vi "InitCell.vi"(6 "Color":u32, 7 "HeadPos":T1, 8 "error in (no error)":errorcluster, 9 "Direction":T2, 10 "CellPosInBody":u16, 11 "Cell":enum16{"Head", "Tail", "Body"}(ring)) -> (0 "error out":errorcluster, 3 "SnakeBodyCell out":refnum<class "SnakeBodyCell.lvclass">)   [LabVIEW 2018, in "SnakeBodyCell.lvclass"]
uses:
  SnakeBodyCell.lvclass
  Typedefs/UnitDirection.ctl
  Typedefs/XYposition.ctl
  SnakeBodyCell.lvclass/SnakeBodyCell.ctl
panel:
  # "Connector Pane"
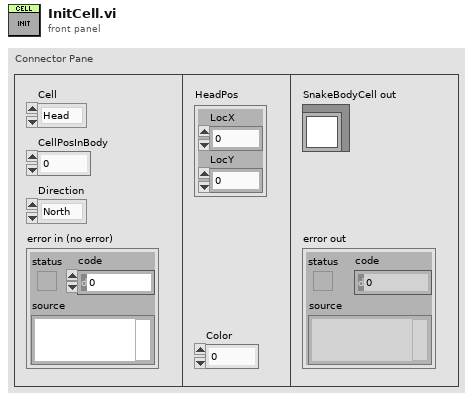
[diagram p1: front panel]
types:
  T1 = typedef "XYposition.ctl" = cluster{"LocX":u16, "LocY":u16}
  T2 = typedef "UnitDirection.ctl" = enum16{"North", "East", "South", "West"}
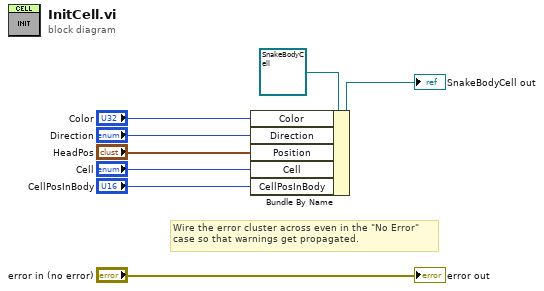
[diagram p0: block diagram]
diagram:
  # "Wire the error cluster across even in the \"No Error\"\ncase so that warnings get propagated."
  n1 = Bundle By Name(cluster=refnum<class "SnakeBodyCell.lvclass"> refnum ("SnakeBodyCell in"), "Color"="Color", "Direction"="Direction", "Position"="HeadPos", "Cell"="Cell", "CellPosInBody"="CellPosInBody") -> (→"SnakeBodyCell out":refnum<class "SnakeBodyCell.lvclass">)
  "error out" <- "error in (no error)"
